vi "DFD Elliptic Design.vi"(4 "ripples [dB]":T1={"passband ripple"=1.0, "stopband atten"=60.0} {"stopband atten" format="%.2f"; "passband ripple" format="%.2f"}, 6 "fs [Hz]":dbl=1.0 format="%.2f", 7 "filter type":T2(ring), 8 "error in (no error)":errorcluster, 9 "low cutoff freq [Hz]":dbl=0.12, 10 "high cutoff freq [Hz]":dbl=0.45, 11 "order":i32=2) -> (0 "error out":errorcluster, 3 "filter out":T3={"mSRate_Fs"=1.0, "mSRate_Version"="2.0", "mSRate_Comments"="", "mSRate_OrgCoef"={"type"=enum."Undefined", "gain"=1.0, "coef a (k)"=[], "coef b (v)"=[]}, "mSRate_CurCoef"={"type"=enum."Undefined", "gain"=1.0, "coef a (k)"=[], "coef b (v)"=[]}, "mSRate_Quantized?"=FALSE, "mSRate_QCoef"={"type"=enum."Undefined", "gain"=1.0, "coef a (k)"=[], "coef b (v)"=[]}, "mSRate_QSettings"=[], "mSRate_Order"=0, "mSRate_Scaling"={"mSRate_ScaleByPowerOf2?"=FALSE, "mSRate_ScaleType"=enum."No Norm"}} {"mSRate_QSettings"."source" items=["Coef a/k"=0, "Coef b/v"=7, "Input"=1, "Output"=2, "Multiplicand"=3, "Product"=4, "Sum"=5, "Delay"=6, "Gain"=8]})   [LabVIEW 2017, in "NI_DigFilterLicensed.lvlib"]
doc: "Creates a digital Elliptic infinite impulse response (IIR) filter."
uses:
  <vilib>/addons/Digital Filter Design/NI_DigFilterLicensed.lvlib
  <vilib>/addons/Digital Filter Design/_Objects.llb/DFD Filter Obj.ctl
  <vilib>/addons/Digital Filter Design/_Objects.llb/DFD Filter Coef.ctl
  <vilib>/addons/Digital Filter Design/_Objects.llb/DFD Filter Structure Type Selector.ctl
  <vilib>/addons/Digital Filter Design/_Objects.llb/dfd_Internal Quantization Settings.ctl
  <vilib>/addons/Digital Filter Design/_Objects.llb/dfd_Internal Quantization Srcs.ctl
  <vilib>/addons/Digital Filter Design/_Objects.llb/DFD Coef Norm Type.ctl
  <vilib>/addons/Digital Filter Design/NI_DigFilter_Design.lvlib
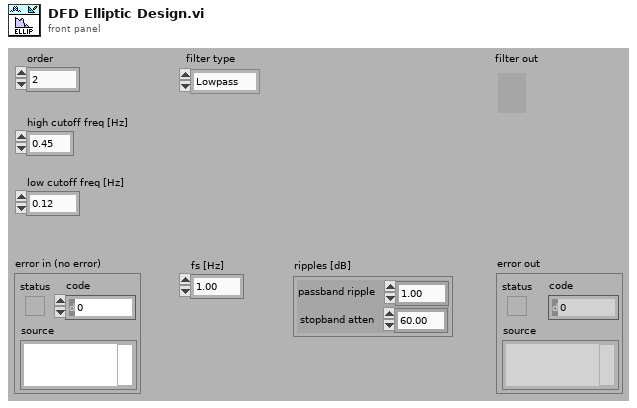
[diagram p1: front panel]
types:
  T1 = cluster{"passband ripple":dbl, "stopband atten":dbl}
  T2 = enum16{"Lowpass", "Highpass", "Bandpass", "Bandstop"}
  T3 = typedef "NI_DigFilterLicensed.lvlib/DFD Filter Obj.ctl" = cluster{"mSRate_Fs":dbl, "mSRate_Version":string, "mSRate_Comments":string, "mSRate_OrgCoef":T4, "mSRate_CurCoef":T4, "mSRate_Quantized?":bool, "mSRate_QCoef":T4, "mSRate_QSettings":T6[], "mSRate_Order":i32, "mSRate_Scaling":cluster{"mSRate_ScaleByPowerOf2?":bool, "mSRate_ScaleType":T8}}
  T4 = typedef "NI_DigFilterLicensed.lvlib/DFD Filter Coef.ctl" = cluster{"type":T5, "gain":dbl, "coef a (k)":dbl[], "coef b (v)":dbl[]}
  T5 = typedef "NI_DigFilterLicensed.lvlib/DFD Filter Structure Type Selector.ctl" = enum16{"Undefined", "FIR Direct Form", "FIR Direct Form Transposed", "FIR Symmetric", "FIR Antisymmetric", "IIR Direct Form I", "IIR Direct Form I Transposed", "IIR Direct Form II", "IIR Direct Form II Transposed", "IIR Cascaded Second Order Sections Form I", "IIR Cascaded Second Order Sections Form I Transposed", "IIR Cascaded Second Order Sections Form II", "IIR Cascaded Second Order Sections Form II Transposed", "Lattice Allpass (basic sections)", "Lattice Allpass (one multiplier sections)", "Lattice Allpass (normalized sections)", "Lattice AR (basic sections)", "Lattice AR (one multiplier sections)", "Lattice AR (normalized sections)", "Lattice MA (minimum phase)", "Lattice MA (maximum phase)", "Lattice ARMA (basic sections)", "Lattice ARMA (one multiplier sections)", "Lattice ARMA (normalized sections)"}
  T6 = typedef "NI_DigFilterLicensed.lvlib/dfd_Internal Quantization Settings.ctl" = cluster{"source":T7, "wl":i16, "iwl":i16, "overflow mode":enum16{"Saturation", "Wrap"}, "rounding mode":enum16{"Nearest", "Truncation"}, "signed?":bool}
  T7 = typedef "NI_DigFilterLicensed.lvlib/dfd_Internal Quantization Srcs.ctl" = u16
  T8 = typedef "NI_DigFilterLicensed.lvlib/DFD Coef Norm Type.ctl" = enum16{"No Norm", "Time Domain 1-Norm", "Time Domain 2-Norm", "Time Domain Inf-Norm"}
  T9 = enum16{"Butterworth", "Chebyshev", "Inv Chebyshev", "Elliptic", "Bessel"}
  T10 = typedef "NI_DigFilterLicensed.lvlib/DFD Pole-Zero.ctl" = cluster{"value":cdb, "z attr":cluster{"real":bool, "lp":bool, "uc":bool}, "order":i32}
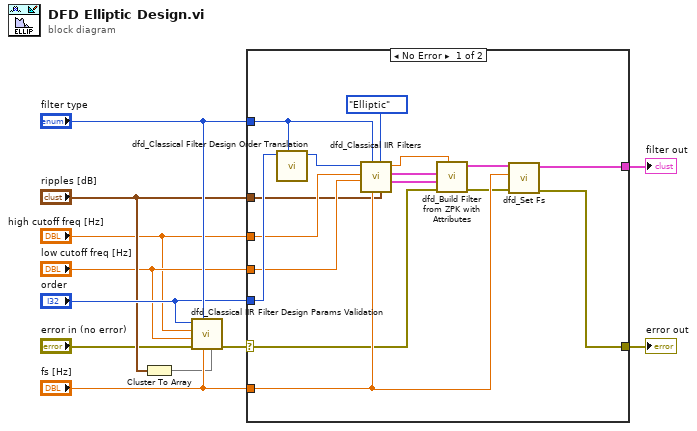
[diagram p0: block diagram]
diagram:
  n1 = Cluster To Array(cluster="ripples [dB]") -> (array=w2:dbl[])
  n2 = call <vilib>:"dfd_Classical IIR Filter Design Params Validation.vi"("params"=w2, "fs [Hz]"="fs [Hz]", "filter type"="filter type", "error in (no error)"="error in (no error)", "low cutoff freq: fl"="low cutoff freq [Hz]", "high cutoff freq: fh"="high cutoff freq [Hz]", "order"="order") -> ("error out"=w1:errorcluster)  [unwired: 4 out]
  n3 = case shown="No Error" w1 {
    selector: w1 -> [w16 w28]
    tunnel: [w13 _] -> w11
    tunnel: [w12 w28] -> w10
    tunnel: "filter type" -> [w27 _]
    tunnel: "order" -> [w26 _]
    tunnel: "ripples [dB]" -> [w15 _]
    tunnel: "fs [Hz]" -> [w25 _]
    tunnel: "low cutoff freq [Hz]" -> [w24 _]
    tunnel: "high cutoff freq [Hz]" -> [w23 _]
    frame No Error {
      n4 = call <vilib>:"dfd_Classical Filter Design Order Translation.vi"("filter type"=w27, "input order"=w26) -> ("order for design"=w19:i32)  [unwired: 9 out]
      n5 = call <vilib>:"dfd_Classical IIR Filters.vi"("ripples [dB]"=w15, "filter design"=T9."Elliptic", "fs [Hz]"=w25, "filter type"=w27, "low cutoff freq: fl"=w24, "high cutoff freq: fh"=w23, "order"=w19) -> ("poles"=w22:T10[], "zeros"=w21:T10[], "gain"=w20:dbl)  [unwired: 1 in, 1 out]
      n6 = call <vilib>:"dfd_Build Filter from ZPK with Attributes.vi"("gain"=w20, "error in (no error)"=w16, "poles"=w22, "zeros"=w21) -> ("error out"=w18:errorcluster, "filter out"=w14:T3)  [unwired: 6 out]
      n7 = call <vilib>:"dfd_Set Fs.vi"("error in (no error)"=w18, "fs [Hz]"=w25, "filter in"=w14) -> ("error out"=w12:errorcluster, "filter out"=w13:T3)  [unwired: 7 out]
    }
    frame Error {
    }
  }
  "filter out" <- w11
  "error out" <- w10
